vi "Page_Source_New_Configurable_VI.vi"(8 "error in (no error)":errorcluster, 11 "AB_RESTfulWebService in":refnum<class "AB_RESTfulWebService.lvclass">) -> (0 "error out":errorcluster, 2 "AB_Source_VI out":refnum<class "AB_Source_VI.lvclass">, 3 "AB_RESTfulWebService out":refnum<class "AB_RESTfulWebService.lvclass">)   [LabVIEW 2020, in "AB_RESTfulWebService.lvclass"]
uses:
  <vilib>/AppBuilder/AB_Classes/RESTful/AB_RESTfulWebService.lvclass
  <vilib>/AppBuilder/AB_Classes/Source/VI/AB_Source_VI.lvclass
  <vilib>/AppBuilder/AB_Classes/Source/RESTfulVI/AB_Source_RESTfulVI.lvclass
  e:/builds/penguin/labview/branches/2020/dev/dist/vi.lib/AppBuilder/AB_Classes/Source/VI/AB_Source_VI.lvclass
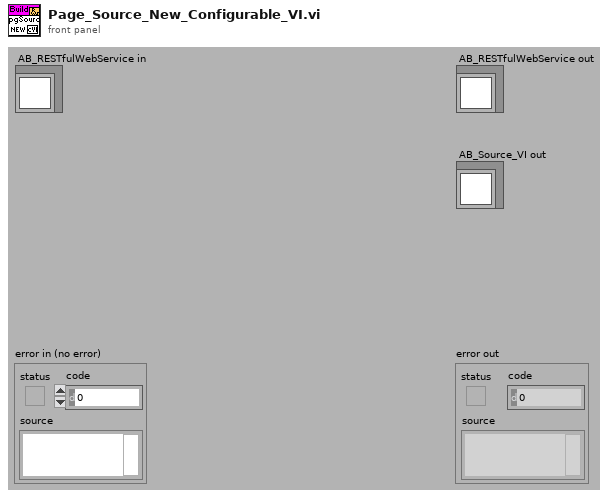
[diagram p1: front panel]
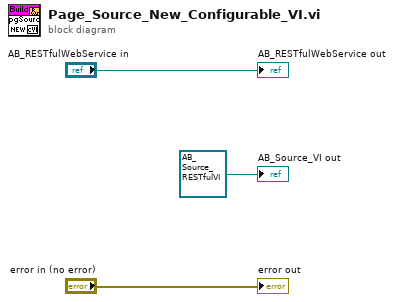
[diagram p0: block diagram]
diagram:
  "error out" <- "error in (no error)"
  "AB_RESTfulWebService out" <- "AB_RESTfulWebService in"
  "AB_Source_VI out" <- refnum<class "AB_Source_RESTfulVI.lvclass"> refnum ("AB_Source_RESTfulVI.lvclass")
